vi "Combine Min Max Vectors.vi"(8 "Other IO Min":dbl[](array[numeric]), 9 "Other IO Max":dbl[](array[numeric]), 10 "IO Min":dbl[](array[numeric]), 11 "IO Max":dbl[](array[numeric])) -> (1 "IO Min":dbl[](array[numeric]), 3 "IO Max":dbl[](array[numeric]))   [LabVIEW 2015, in "Teaching File.lvlib"]
uses:
  Teaching File.lvlib
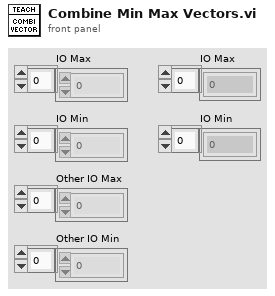
[diagram p1: front panel]
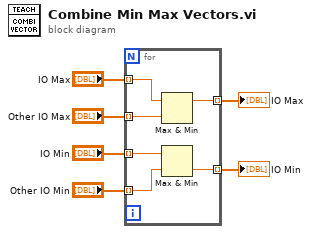
[diagram p0: block diagram]
diagram:
  n1 = for {
    tunnel: "IO Min" -> [w10] mode=indexing
    tunnel: "Other IO Min" -> [w9] mode=indexing
    tunnel: "IO Max" -> [w12] mode=indexing
    tunnel: "Other IO Max" -> [w11] mode=indexing
    tunnel: [w8] -> w1 mode=indexing
    tunnel: [w7] -> w2 mode=indexing
    n2 = Max & Min(x=w12, y=w11) -> (max(x,y)=w7:dbl)  [unwired: 1 out]
    n3 = Max & Min(x=w10, y=w9) -> (min(x,y)=w8:dbl)  [unwired: 1 out]
  }
  "IO Max" <- w2
  "IO Min" <- w1
